vi "Configure.vi"(8 "error in (no error)":errorcluster, 9 "Buffer":string, 10 "Function":T1, 11 "Measure in":refnum<class "Measure.lvclass">) -> (0 "error out":errorcluster, 3 "Measure out":refnum<class "Measure.lvclass">)   [LabVIEW 2023, in "HAF.lvlib" / "Measure.lvclass"]
doc: "Set up the Measurement Command with a Function and Buffer."
uses:
  Measure.lvclass
  Measure Function.ctl
  HAF.lvlib
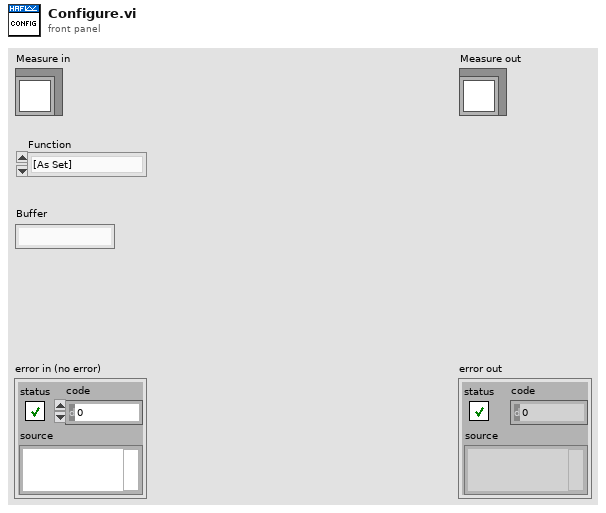
[diagram p1: front panel]
types:
  T1 = typedef "HAF.lvlib/Measure Function.ctl" = enum16{"[As Set]", "DC Voltage", "AC Voltage", "DC Current", "AC Current", "2-wire Resistance", "4-wire Resistance", "Diode", "Capacitance", "Temperature", "Continuity", "Frequency", "Period", "DC Voltage Ratio"}
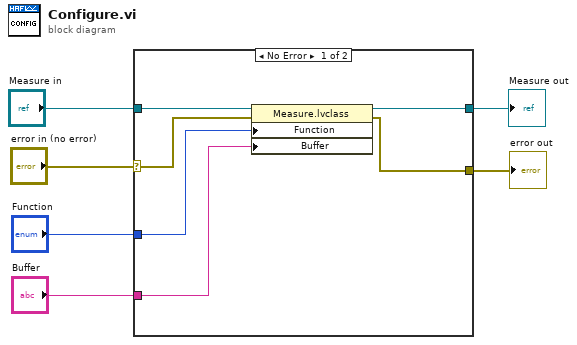
[diagram p0: block diagram]
diagram:
  n1 = case shown="No Error" "error in (no error)" {
    selector: "error in (no error)" -> [w10 w14]
    tunnel: [w7 w14] -> w5
    tunnel: [w11 w13] -> w3
    tunnel: "Measure in" -> [w12 w13]
    tunnel: "Function" -> [w9 _]
    tunnel: "Buffer" -> [w8 _]
    frame No Error {
      n2 = property class="Measure.lvclass"(reference=w12, error in=w10, "Function"=w9, "Buffer"=w8) -> (reference out=w11:refnum<class "Measure.lvclass">, error out=w7:errorcluster)
    }
    frame Error {
    }
  }
  "error out" <- w5
  "Measure out" <- w3
